vi "Lockin Engine.vi"(8 "error in (no error)":errorcluster, 11 "Lockin.DAQ":refnum<class "Instrument.DAQ.lvclass">) -> (0 "error out":errorcluster, 1 "SweepResults":T1, 2 "<Results> (X,Y,R,Theta,Mean)":T2 {"Results (Dictionary)"."value" format="%#_6p"}, 3 "Lockin.DAQ":refnum<class "Instrument.DAQ.lvclass">)   [LabVIEW 2019, in "Instrument.DAQ.lvclass"]
uses:
  Instrument.DAQ.lvclass
  Typedefs/Results--Cluster.ctl
  <vilib>/Analysis/NI_AALBase.lvlib
  <vilib>/Analysis/baseanly.llb/Mean (DBL).vi
panel:
  out "Y Results":cluster{i32[], dbl[]}[](graph)
  out "X Results":cluster{i32[], dbl[]}[](graph)
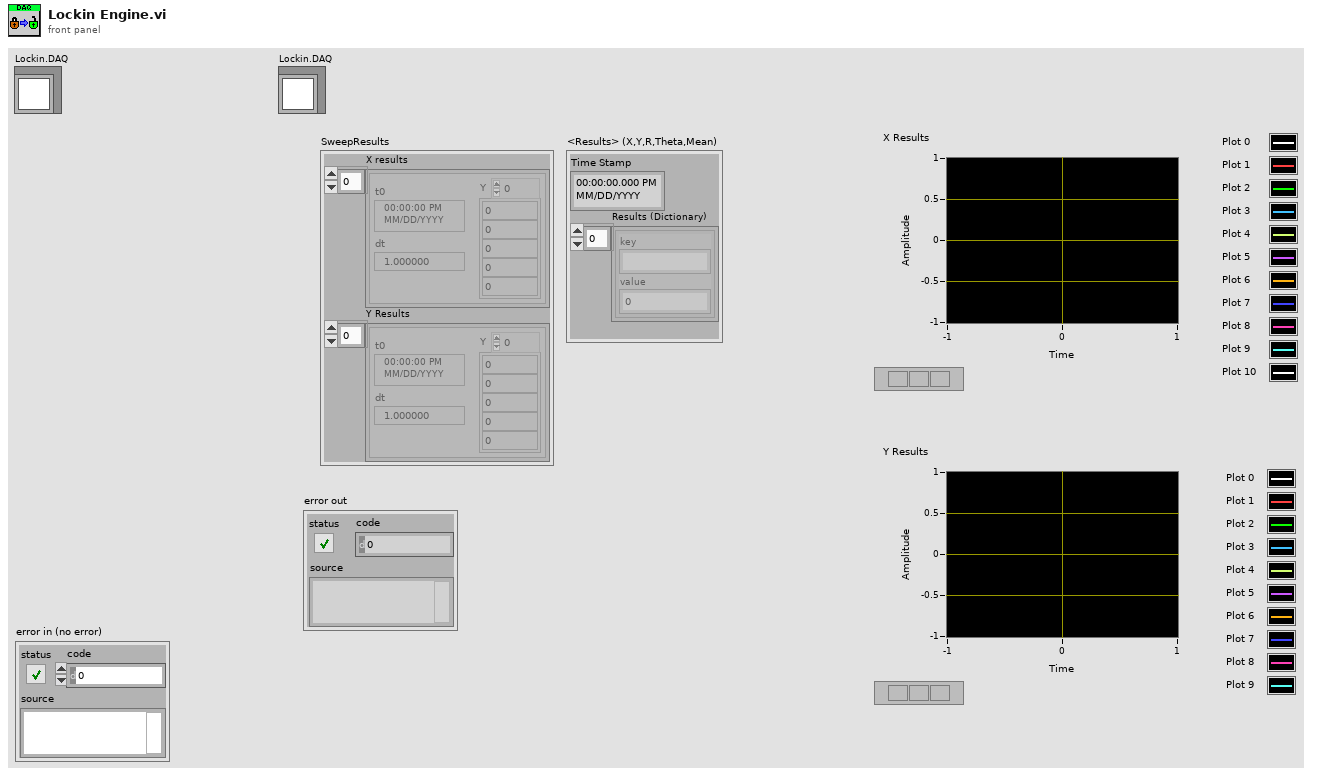
[diagram p1: front panel]
types:
  T1 = cluster{"X results":waveform(dbl)[], "Y Results":waveform(dbl)[]}
  T2 = typedef "Instrument.DAQ.lvclass/Results--Cluster.ctl" = cluster{"Time Stamp":timestamp, "Results (Dictionary)":cluster{"key":string, "value":dbl}[]}
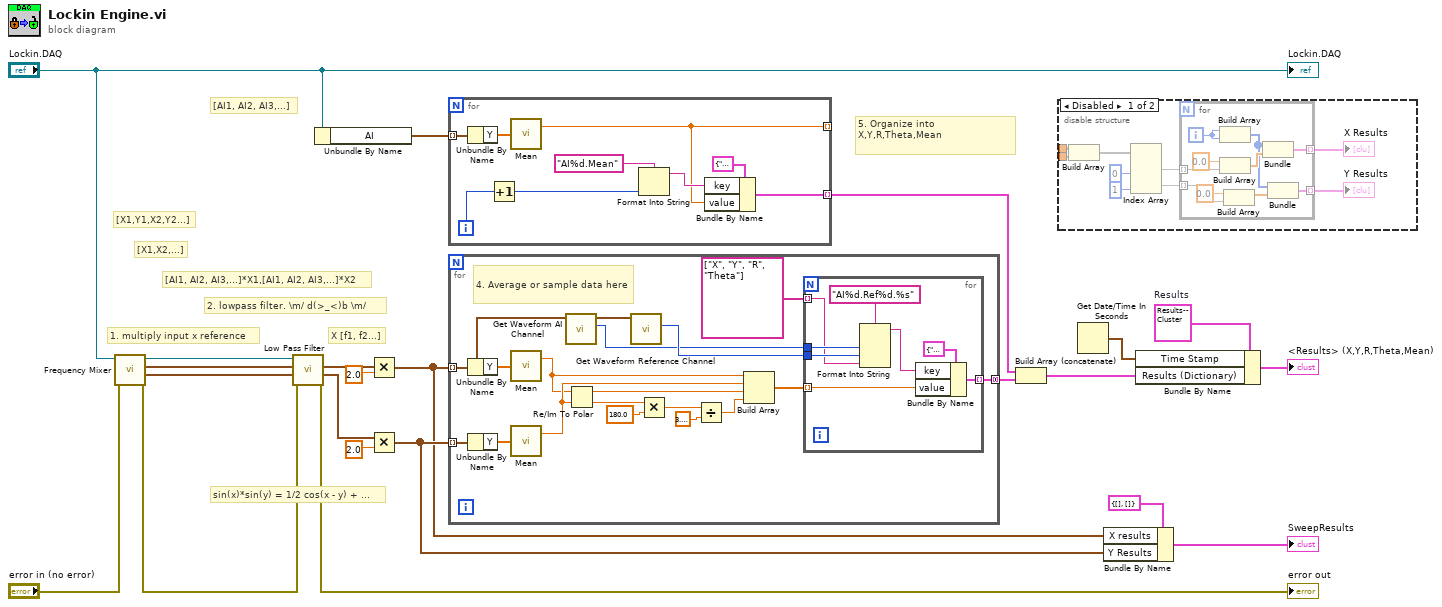
[diagram p0: block diagram]
diagram:
  w22 = T2 {"Time Stamp"=timestamp(0 s since 1904-01-01), "Results (Dictionary)"=[]}  # Results
  # "sin(x)*sin(y) = 1/2 cos(x - y) + ..."
  # "[X1,X2,...]"
  # "1. multiply input x reference"
  # "X [f1, f2...]"
  # "2. lowpass filter. \\m/ d(>_<)b \\m/"
  # "[AI1, AI2, AI3,...]*X1,[AI1, AI2, AI3,...]*X2"
  # "[AI1, AI2, AI3,...]"
  # "[X1,Y1,X2,Y2...]"
  # "5. Organize into X,Y,R,Theta,Mean"
  n1 = call "Frequency Mixer.vi"("error in (no error)"="error in (no error)", "Lockin.DAQ"="Lockin.DAQ") -> ("error out"=w15:errorcluster, "Y"=w4:waveform(dbl)[], "X"=w16:waveform(dbl)[], "Lockin.DAQ"=w20:refnum<class "Instrument.DAQ.lvclass">)  [unwired: 6 in]
  n2 = call "Low Pass Filter.vi"("error in (no error)"=w15, "Y"=w4, "X"=w16, "Lockin.DAQ"=w20) -> ("error out"=→"error out":errorcluster, "Y 2"=w2:waveform(dbl)[], "X 2"=w3:waveform(dbl)[])  [unwired: 4 in, 1 out]
  n3 = Unbundle By Name("Lockin.DAQ") -> ("AI"=w5:waveform(dbl)[])
  n4 = Multiply(x=w3, y=2.0) -> (x*y=w11:waveform(dbl)[])
  n5 = Multiply(x=w2, y=2.0) -> (x*y=w12:waveform(dbl)[])
  n6 = for {
    tunnel: w5 -> [w31] mode=indexing
    tunnel: [w26] -> _ mode=indexing
    tunnel: [w25] -> w8 mode=indexing
    i -> [w24]
    n7 = Unbundle By Name(w31) -> ("Y"=w30:dbl[])
    n8 = Increment(x=w24) -> (x+1=w23:i32)
    n9 = call-poly <vilib>:"Mean.vi"("X"=w30) -> ("mean"=w26:dbl)  [unwired: 1 out]
    n10 = Format Into String(format string="AI%d.Mean", w23) -> (resulting string=w28:string)  [unwired: 2 in, 1 out]
    n11 = Bundle By Name(cluster=cluster{"key":string, "value":dbl} {"key"="", "value"=0.0} ("key-value"), "key"=w28, "value"=w26) -> (w25:cluster{"key":string, "value":dbl})
  }
  n12 = for {
    tunnel: w11 -> [w38] mode=indexing
    tunnel: w12 -> [w40] mode=indexing
    tunnel: [w35] -> w9 mode=concatenating
    # "4. Average or sample data here"
    n13 = Unbundle By Name(w38) -> ("Y"=w43:dbl[])
    n14 = Unbundle By Name(w40) -> ("Y"=w42:dbl[])
    n15 = call-poly <vilib>:"Mean.vi"("X"=w43) -> ("mean"=w39:dbl)  [unwired: 1 out]
    n16 = call-poly <vilib>:"Mean.vi"("X"=w42) -> ("mean"=w41:dbl)  [unwired: 1 out]
    n17 = call "Get Waveform AI Channel.vi"("Reference in"=w38) -> ("AI Channel"=w32:u16, "Reference out"=w37:waveform(dbl))  [unwired: 8 in, 1 out]
    n18 = Re/Im To Polar(2:w41, 3:w39) -> (0:w46:dbl, 1:w44:dbl)
    n19 = call "Get Waveform Reference Channel.vi"("Reference in"=w37) -> ("Reference Channel"=w33:u16)  [unwired: 8 in, 2 out]
    n20 = Multiply(x=w46, y=180.0) -> (x*y=w45:dbl)
    n21 = Divide(x=w45, y=3.141592653589793) -> (x/y=w49:dbl)
    n22 = Build Array(w39, w41, w44, w49) -> (w34:dbl[])
    n23 = for {
      tunnel: w34 -> [w57] mode=indexing
      tunnel: string[] ["X", "Y", "R", "Theta"] -> [w51] mode=indexing
      tunnel: [w55] -> w35 mode=indexing
      tunnel: w33 -> [w52]
      tunnel: w32 -> [w54]
      n24 = Format Into String(format string="AI%d.Ref%d.%s", w54, w52, w51) -> (resulting string=w50:string)  [unwired: 2 in, 1 out]
      n25 = Bundle By Name(cluster=cluster{"key":string, "value":dbl} {"key"="", "value"=0.0} ("key-value"), "key"=w50, "value"=w57) -> (w55:cluster{"key":string, "value":dbl})
    }
  }
  n26 = Build Array (concatenate)(w8, w9) -> (w7:cluster{"key":string, "value":dbl}[])
  n27 = disable-structure shown="Disabled" {
    disable-tunnel: _ -> [w60 _]
    disable-tunnel: _ -> [w59 _]
    frame Disabled {
      n28 = Build Array(w59, w60) -> (w58:void[])
      n29 = Index Array(array=w58, index (col) #1=0 ("disabled index (col)"), index (col) #2=1 ("index (col)")) -> (element #1=w66:void[], element #2=w62:void[])  [unwired: 2 in]
      n30 = for {
        tunnel: w66 -> [w76] mode=indexing
        tunnel: [w74] -> w65 mode=indexing
        tunnel: w62 -> [w68] mode=indexing
        tunnel: [w67] -> w61 mode=indexing
        i -> [w73]
        n31 = Build Array(w73, w73) -> (w70:i32[])
        n32 = Build Array(0.0 ("element"), w76) -> (w72:dbl[])
        n33 = Build Array(0.0 ("element"), w68) -> (w69:dbl[])
        n34 = Bundle(w70, w72) -> (w74:cluster{i32[], dbl[]})  [unwired: 1 in]
        n35 = Bundle(w70, w69) -> (w67:cluster{i32[], dbl[]})  [unwired: 1 in]
      }
      "X Results" <- w65
      "Y Results" <- w61
    }
    frame Enabled {
    }
  }
  n36 = Get Date/Time In Seconds() -> (seconds since 1Jan1904=w1:timestamp)
  n37 = Bundle By Name(cluster=T1 {"X results"=[], "Y Results"=[]} ("SweepResults"), "X results"=w11, "Y Results"=w12) -> (→"SweepResults":T1)
  n38 = Bundle By Name(cluster=w22, "Time Stamp"=w1, "Results (Dictionary)"=w7) -> (→"<Results> (X,Y,R,Theta,Mean)":T2)
  "Lockin.DAQ" <- "Lockin.DAQ"
